vi "PH_HamamatsuCamera.State On.vi"(0 "VI in":refnum<vi>, 1 "Cam Handle in":i32, 4 "Cam Error in":errorcluster {"code" format="%.0x"}, 5 "error in (no error)":errorcluster) -> (14 "VI out":refnum<vi>, 15 "Cam Handle":i32, 18 "Cam Error":errorcluster, 19 "error out":errorcluster)   [LabVIEW 2014, in "PH_HamamatsuCamera.lvlib"]
uses:
  PH_HamamatsuCamera.lvlib
  PH_Cam_BaseClass/PH_Cam_BaseClass.lvlib
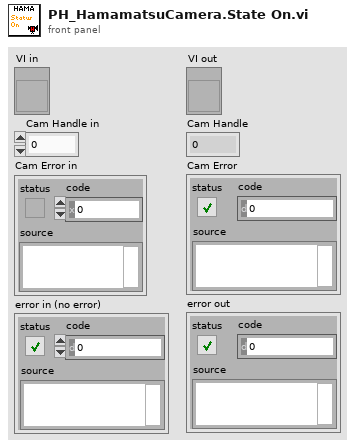
[diagram p1: front panel]
types:
  T1 = typedef "PH_HamamatsuCamera.lvlib/PH_HamamatsuCamera.i attribute.ctl" = cluster{"Gui Refs":cluster{"Camera Details":refnum<vi>, "ROI":refnum<vi>, "Set ROI to Maximum":refnum<vi>, "Trigger Parameters":refnum<vi>, "Brightness":refnum<vi>, "Shutter":refnum<vi>, "Gain":refnum<vi>, "Trigger Timeout":refnum<vi>, "Trigger Polarity":refnum<vi>, "Trigger Mode":refnum<vi>, "Parameters":refnum<vi>, "Set Cam Parameter":refnum<vi>, "Parameter to set":refnum<vi>, "Value to set":refnum<vi>}, "Cam":cluster{"Handle":i32, "Details":cluster{"Model":string, "Camera ID":string, "Firmware":string}, "Buffer Info":cluster{"height":u32, "width":u32, "datatype":u32}}, "H Offset":cluster{"Value":i32, "Minimum":i32, "Maximum":i32, "Increment":i32}, "V Offset":cluster{"Value":i32, "Minimum":i32, "Maximum":i32, "Increment":i32}, "H Width":cluster{"Value":i32, "Minimum":i32, "Maximum":i32, "Increment":i32}, "V Width":cluster{"Value":i32, "Minimum":i32, "Maximum":i32, "Increment":i32}, "Trigger Parameters":T2, "Trigger Timeout":u32, "Parameters":T3[], "Indicees Cam Parameters":cluster{"Brightness":i32, "Shutter":i32, "Gain":i32}, "Wanted Values":cluster{"Trigger Settings":T2[], "ROI":T4[], "Parameter":cluster{"Name":string, "Value":dbl}[]}}
  T2 = typedef "PH_HamamatsuCamera.lvlib/PH_HamamatsuCamera.Trigger Parameter.ctl" = cluster{"Mode":u32, "Polarity":u32, "Times":u32, "Delay":dbl}
  T3 = typedef "PH_HamamatsuCamera.lvlib/PH_HamamatsuCamera.Parameter Set.ctl" = cluster{"Parameter":string, "Value":dbl, "Writable":bool, "Range":cluster{"min":dbl, "max":dbl, "step":dbl}, "Default":dbl, "Value Names":cluster{"Name":string, "Value":dbl}[], "Text Values":bool}
  T4 = typedef "PH_HamamatsuCamera.lvlib/PH_HamamatsuCamera.ROI.ctl" = cluster{"Horizontal Offset":i32, "Vertical Offset":i32, "Horizontal Width":i32, "Vertical Width":i32}
  T5 = cluster{"height":u32, "width":u32, "datatype":u32}
  T6 = typedef "PH_Cam_BaseClass.lvlib/PH_Cam_BaseClass.i attribute.ctl" = cluster{"Gui Refs":T7, "Cam":cluster{"Source Notifier":refnum<notifier>, "Error":errorcluster, "Camera ID":string}, "Images":cluster{"Cam":T8, "Operation":T8, "PSDB":T8}, "Window Image":cluster{"Indicate Image":bool, "Window No.":i32, "Scale Facor":dbl, "Center Cross":bool, "Subtract Backgr":bool, "CoG":bool, "Color Palette":cluster{"Red":u8, "Green":u8, "Blue":u8}[], "Image On":bool}, "Default Prdc Int":i32, "Performance":cluster{"on":bool, "Timestamp Last Frame":i32}, "Histogram":cluster{"on":bool, "Mapping":bool}, "Save Image":cluster{"Save":bool, "File refnum":refnum<file>}, "Setting Service ID":i32, "Screen":cluster{"x-resolution":i16, "y-resolution":i16}, "On":bool, "Constructor finished":bool, "configured":bool}
  T7 = typedef "PH_Cam_BaseClass.lvlib/PH_Cam_BaseClass.GUI Refs.ctl" = cluster{"Frame Rate":refnum<vi>, "Get Frame Rate":refnum<vi>, "Show Image":refnum<vi>, "Get Histogram":refnum<vi>, "Mapping":refnum<vi>, "Histogram":refnum<vi>, "Center Cross":refnum<vi>, "Center of Gravity":refnum<vi>, "Scale Factor [%]":refnum<vi>, "Save Image":refnum<vi>, "Palette":refnum<vi>, "Subtract Background":refnum<vi>, "Cam Error":refnum<vi>, "On":refnum<vi>, "Cam List":refnum<vi>}
  T8 = typedef "IMAQ Image.ctl" = refnum<image>
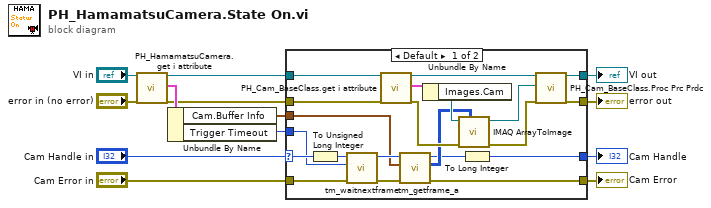
[diagram p0: block diagram]
diagram:
  n1 = call "PH_HamamatsuCamera.get i attribute.vi"("i ref in"="VI in", "error in (no error)"="error in (no error)") -> ("i ref out"=w13:refnum<vi>, "i attribute"=w12:T1, "error out"=w11:errorcluster)  [unwired: 15 in]
  n2 = Unbundle By Name(w12) -> ("Cam.Buffer Info"=w9:T5, "Trigger Timeout"=w10:u32)
  n3 = case shown="Default" "Cam Handle in" {
    selector: "Cam Handle in" -> [w34 w36]
    tunnel: w11 -> [w19 w38]
    tunnel: [w25 w38] -> w8
    tunnel: w13 -> [w20 w37]
    tunnel: [w26 w37] -> w7
    tunnel: w10 -> [w32 _]
    tunnel: w9 -> [w29 _]
    tunnel: [w17 w35] -> w3
    tunnel: [w15 w36] -> w2
    tunnel: "Cam Error in" -> [w14 w35]
    frame Default {
      n4 = To Unsigned Long Integer(number=w34) -> (unsigned 32bit integer=w33:u32)
      n5 = call <userlib>:"tm_waitnextframe.vi"("error in (no error)"=w14, "Timeout"=w32, "Handle in"=w33) -> ("error out"=w30:errorcluster, "Handle out"=w31:u32)  [unwired: 5 in, 2 out]
      n6 = call "PH_Cam_BaseClass.get i attribute.vi"("i ref in"=w20, "error in (no error)"=w19) -> ("i ref out"=w27:refnum<vi>, "i attribute"=w28:T6, "error out"=w23:errorcluster)  [unwired: 15 in]
      n7 = call <userlib>:"tm_getframe_a.vi"("error in (no error)"=w30, "Buffer Info"=w29, "Handle in"=w31) -> ("error out"=w17:errorcluster, "Data 16"=w18:u16[][], "Handle out"=w16:u32)  [unwired: 4 in, 2 out]
      n8 = Unbundle By Name(w28) -> ("Images.Cam"=w24:T8)
      n9 = call "IMAQ ArrayToImage"("Image Pixels (U16)"=w18, "error in (no error)"=w23, "Image"=w24) -> ("error out"=w22:errorcluster, "Image Out"=w21:T8)  [unwired: 7 in]
      n10 = To Long Integer(number=w16) -> (32bit integer=w15:i32)
      n11 = call "PH_Cam_BaseClass.Proc Prc Prdc.vi"("VI in"=w27, "Image In"=w21, "error in (no error)"=w22) -> ("VI out"=w26:refnum<vi>, "error out"=w25:errorcluster)  [unwired: 15 in]
    }
    frame -1 {
    }
  }
  "Cam Error" <- w3
  "error out" <- w8
  "VI out" <- w7
  "Cam Handle" <- w2
